vi "test_DiscoveryServiceNotRunning_LaunchDiscoveryService_DiscoveryServiceStarted.vi"(8 "error in":errorcluster) -> (0 "error out":errorcluster, 2 "result":string, 3 "pass":bool)   [LabVIEW 2020, in "MeasurementServerTests.lvlib" / "Discovery Tests.lvlib"]
uses:
  Discovery Tests.lvlib
  Runtime/MeasurementLink Discovery V1/MeasurementLink Discovery V1.lvlib
  MeasurementServerTests.lvlib
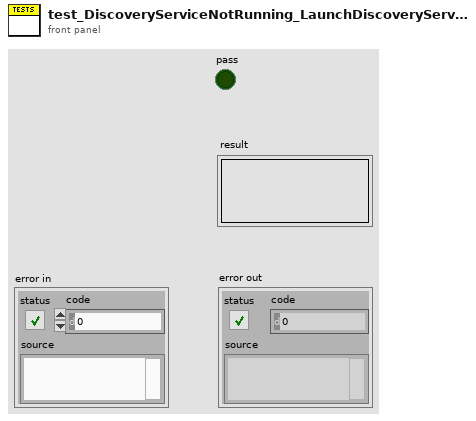
[diagram p1: front panel]
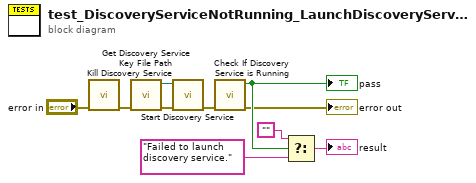
[diagram p0: block diagram]
diagram:
  n1 = call "Kill Discovery Service.vi"("error in"="error in") -> ("error out"=w8:errorcluster)  [unwired: 10 in]
  n2 = call "Get Discovery Service Key File Path.vi"("error in"=w8) -> ("error out"=w10:errorcluster, "key file path"=w4:path)  [unwired: 9 in]
  n3 = call "Start Discovery Service.vi"("error in"=w10, "key file path"=w4) -> ("error out"=w3:errorcluster)  [unwired: 9 in]
  n4 = call "Check If Discovery Service is Running.vi"("error in (no error)"=w3) -> ("error out"=→"error out":errorcluster, "discovery service running?"=w2:bool)  [unwired: 9 in]
  "pass" <- w2
  n5 = Select(t="", s=w2, f="Failed to launch discovery service.") -> (s? t:f=→"result":string)
